vi "Lab Panel V5.28.vi"() -> ()   [LabVIEW 2013] (continued)
                                n843 = Unbundle(w1484) -> ("DESCRIPTION"=w1483:string)  [unwired: 4 out]
                                n844 = Concatenate Strings(w1479, "\\", w1477, w1475, w1476, w1475) -> (w1486:string)
                                n845 = String To Path(string=w1486) -> (path=w1488:path)
                                n846 = Concatenate Strings(w1486, w1485, w1483, "-", w1482, ".tdms") -> (w1474:string)
                                n847 = Create Folder(path (use dialog)=w1488) -> (error out=w1487:errorcluster)  [unwired: 2 in, 2 out]
                                n848 = global write "Global 1.vi" "LAB03-2 FILE"(w1474) -> ()
                                n849 = call <vilib>:"Clear Errors.vi"("error in (no error)"=w1487) -> ()  [unwired: 6 in, 1 out]
                              }
                              frame #1 {
                                (unwired) FALSE
                                n850 = String To Path(string=w1498) -> (path=w1494:path)
                                n851 = TDMS Open(6:FALSE, 10:T21."create or replace" ("operation (0:open)"), 11:w1494) -> (0:w1493:errorcluster, 3:→"TDMS LAB03-2":refnum<k34>)  [unwired: 4 in]
                              }
                              frame #2 {
                                n852 = local read "SET LAB03-2"() -> (w1504:T5)
                                n853 = local read "TDMS LAB03-2"() -> (w1515:refnum<k34>)
                                n854 = Build Array("Testers Name", "Description", "Set Test Cycles", "T-Rise minutes", "T-Rise Deg C") -> (w1505:string[])
                                n855 = Unbundle(w1504) -> ("NAME"=w1503:string, "DESCRIPTION"=w1502:string, "CYCLES"=w1501:dbl, "T-RISE mins"=w1500:dbl, "T-RISE deg C"=w1499:dbl)
                                n856 = Number To Decimal String(number=w1501) -> (decimal integer string=w1514:string)  [unwired: 1 in]
                                n857 = Number To Decimal String(number=w1500) -> (decimal integer string=w1513:string)  [unwired: 1 in]
                                n858 = Number To Decimal String(number=w1499) -> (decimal integer string=w1512:string)  [unwired: 1 in]
                                n859 = Build Array(w1503, w1502, w1514, w1513, w1512) -> (w1511:string[])
                                n860 = TDMS Set Properties(5:w1511, 7:w1505, 11:w1515) -> ()  [unwired: 3 in, 4 out]
                              }
                              frame #3 {
                                n861 = local read "DISP LAB03-2"() -> (w1520:T4)
                                n862 = Concatenate Strings("LAB03-2  ", w1519) -> (w1521:string)
                                n863 = Two Button Dialog(message=w1521, 1:w1517, 2:w1518) -> (T button?=w1523:bool)
                                n864 = case shown="True" w1523 {
                                tunnel: w1520 -> [w1530 w1531]
                                tunnel: [w1530 w1531] -> w1527
                                tunnel: [w1529 w1532] -> w1526
                                tunnel: [w1528 w1532] -> w1525
                                frame False {
                                n865 = Unbundle(w1530) -> ("CYCLE"=w1529:dbl, "MINS"=w1528:dbl)  [unwired: 1 out]
                                }
                                frame True {
                                w1532 = 0.0
                                }
                                }
                                n866 = Bundle(cluster=w1527, "CYCLE"=w1526, "MINS"=w1525, "STATUS"="RUN") -> (w1516:T4)
                                n867 = local write "DISP LAB03-2"(w1516) -> ()
                              }
                              frame #4 {
                                n868 = local read "TEMP START LAB03-2"() -> (w1535:cluster{"TL":dbl, "TN":dbl})
                                n869 = Bundle(cluster=w1535, "TL"=w1533, "TN"=w1533) -> (w1534:cluster{"TL":dbl, "TN":dbl})
                                n870 = local write "TEMP START LAB03-2"(w1534) -> ()
                              }
                            }
                          }
                        }
                      }
                    }
                  }
                }
              }
              event "RUN LAB04-1": Value Change {
                n871 = event-data() -> ("NewVal"=w1540:bool)  [unwired: 1 in, 5 out]
                n872 = local write "run lab04-1"(w1540) -> ()
                n873 = case shown="True" w1540 {
                  tunnel: w1546 -> [_ w1584]
                  tunnel: w1545 -> [_ w1583]
                  tunnel: w1543 -> [w1548 w1582]
                  tunnel: w1544 -> [_ w1581]
                  tunnel: w1542 -> [_ w1580]
                  tunnel: [w1547 w1579] -> w1541
                  tunnel: w1539 -> [_ w1578]
                  tunnel: w1538 -> [_ w1577]
                  tunnel: w1537 -> [_ w1576]
                  tunnel: w1536 -> [_ w1574]
                  frame False {
                    # "stop test"
                    n874 = stacked-sequence {
                      tunnel: w1548 -> [w1557 _]
                      tunnel: [w1549 _] -> w1547
                      frame #0 {
                        n875 = local read "DISP LAB04-1"() -> (w1556:T4)
                        n876 = Unbundle(w1556) -> ("CYCLE"=w1554:dbl, "MINS"=w1555:dbl)  [unwired: 1 out]
                        n877 = case shown="\"CYCLE TEST\"" w1557 {
                          tunnel: w1555 -> [_ _ w1564]
                          tunnel: w1554 -> [w1562 w1563 _]
                          tunnel: [w1562 w1563 w1564] -> w1553
                          frame "CHART TEST", Default {
                          }
                          frame "CYCLE TEST" {
                          }
                          frame "T-RISE TEST" {
                          }
                        }
                        n878 = local read "TDMS LAB04-1"() -> (w1561:refnum<k34>)
                        n879 = Build Array("STOPPED") -> (w1558:string[])
                        n880 = Build Array(w1553) -> (w1552:dbl[])
                        n881 = TDMS Write(0:w1561, 5:"TEST RESULT", 7:w1558, 9:w1552) -> (4:w1550:refnum<k34>, 15:w1551:errorcluster)  [unwired: 2 in, 2 out]
                        n882 = TDMS Close(8:w1551, 11:w1550) -> (0:w1549:errorcluster)  [unwired: 1 out]
                      }
                      frame #1 {
                        n883 = local read "DISP LAB04-1"() -> (w1568:T4)
                        n884 = stacked-sequence {
                          tunnel: "LAB04-1" -> [w1570 w1572]
                          frame #0 {
                            n885 = call "sub vi - defrag tdms v1.vi"("panel id"=w1570) -> ("error out"=w1569:errorcluster)  [unwired: 10 in]
                            n886 = local write "data file error"(w1569) -> ()
                          }
                          frame #1 {
                            n887 = call "Save data file (stop) v3.vi"("panel id"=w1572) -> ("network file save error"=w1571:errorcluster)  [unwired: 9 in, 1 out]
                            n888 = local write "RESULT LAB04-1"(FALSE) -> ()
                            n889 = local write "data file error"(w1571) -> ()
                          }
                        }
                        n890 = Bundle(cluster=w1568, "STATUS"="STOP") -> (w1566:T4)  [unwired: 2 in]
                        n891 = local write "DISP LAB04-1"(w1566) -> ()
                      }
                    }
                  }
                  frame True {
                    n892 = local read "SIG LAB04-1"() -> (w1575:T2)
                    n893 = stacked-sequence {
                      seq-local: [w1586 _] -> [_ w1590]
                      tunnel: w1584 -> [_ w1600]
                      tunnel: w1583 -> [_ w1599]
                      tunnel: w1582 -> [_ w1598]
                      tunnel: w1581 -> [_ w1597]
                      tunnel: w1580 -> [_ w1596]
                      tunnel: [_ w1595] -> w1579
                      tunnel: w1578 -> [_ w1594]
                      tunnel: w1577 -> [_ w1593]
                      tunnel: w1576 -> [_ w1592]
                      tunnel: w1575 -> [w1585 w1591]
                      tunnel: w1574 -> [_ w1589]
                      frame #0 {
                        n894 = Unbundle(w1585) -> ("AMPS"=w1588:dbl)  [unwired: 4 out]
                        n895 = call "Check For Amps on v1.vi"("ID"="LAB04-1", "amps"=w1588) -> ("amps"=w1586:bool)  [unwired: 9 in]
                      }
                      frame #1 {
                        n896 = case shown="True" w1590 {
                          tunnel: w1600 -> [_ w1613]
                          tunnel: w1599 -> [_ w1612]
                          tunnel: w1598 -> [_ w1611]
                          tunnel: w1597 -> [_ w1610]
                          tunnel: w1596 -> [_ w1609]
                          tunnel: [errorcluster {"status"=FALSE, "code"=0, "source"=""} ("error out") w1608] -> w1595
                          tunnel: w1594 -> [_ w1607]
                          tunnel: w1593 -> [_ w1606]
                          tunnel: w1592 -> [_ w1605]
                          tunnel: w1591 -> [_ w1604]
                          tunnel: w1589 -> [_ w1603]
                          frame False {
                            w1601 = FALSE
                            n897 = local write "RUN LAB04-1"(w1601) -> ()
                            n898 = local write "run lab04-1"(w1601) -> ()
                          }
                          frame True {
                            n899 = stacked-sequence {
                              seq-local: [w1614 _ _ _ _] -> [_ w1638 _ _ _]
                              tunnel: w1613 -> [w1619 _ _ _ _]
                              tunnel: w1612 -> [w1615 _ _ _ _]
                              tunnel: w1611 -> [w1629 _ _ _ _]
                              tunnel: w1610 -> [w1622 _ _ _ _]
                              tunnel: w1609 -> [w1617 _ _ _ _]
                              tunnel: [_ w1633 _ _ _] -> w1608
                              tunnel: w1607 -> [_ _ _ w1659 _]
                              tunnel: w1606 -> [_ _ _ w1658 _]
                              tunnel: w1605 -> [_ _ _ w1657 _]
                              tunnel: w1604 -> [_ _ _ _ _]
                              tunnel: w1603 -> [_ _ _ _ w1673]
                              frame #0 {
                                w1616 = "\\"
                                n900 = local read "SET LAB04-1"() -> (w1624:T5)
                                n901 = case shown="\"CYCLE TEST\"" w1629 {
                                tunnel: ["L04-1-CHART TEST-" "L04-1-CYCLE TEST-" "L04-1-T-RISE TEST-"] -> w1625
                                frame "CHART TEST", Default {
                                }
                                frame "CYCLE TEST" {
                                }
                                frame "T-RISE TEST" {
                                }
                                }
                                n902 = Unbundle(w1624) -> ("DESCRIPTION"=w1623:string)  [unwired: 4 out]
                                n903 = Concatenate Strings(w1619, "\\", w1617, w1616, w1615, w1616) -> (w1626:string)
                                n904 = String To Path(string=w1626) -> (path=w1628:path)
                                n905 = Concatenate Strings(w1626, w1625, w1623, "-", w1622, ".tdms") -> (w1614:string)
                                n906 = Create Folder(path (use dialog)=w1628) -> (error out=w1627:errorcluster)  [unwired: 2 in, 2 out]
                                n907 = global write "Global 1.vi" "LAB04-1 FILE"(w1614) -> ()
                                n908 = call <vilib>:"Clear Errors.vi"("error in (no error)"=w1627) -> ()  [unwired: 6 in, 1 out]
                              }
                              frame #1 {
                                (unwired) FALSE
                                n909 = String To Path(string=w1638) -> (path=w1634:path)
                                n910 = TDMS Open(6:FALSE, 10:T21."create or replace" ("operation (0:open)"), 11:w1634) -> (0:w1633:errorcluster, 3:→"TDMS LAB04-1":refnum<k34>)  [unwired: 4 in]
                              }
                              frame #2 {
                                n911 = local read "SET LAB04-1"() -> (w1644:T5)
                                n912 = local read "TDMS LAB04-1"() -> (w1655:refnum<k34>)
                                n913 = Build Array("Testers Name", "Description", "Set Test Cycles", "T-Rise minutes", "T-Rise Deg C") -> (w1645:string[])
                                n914 = Unbundle(w1644) -> ("NAME"=w1643:string, "DESCRIPTION"=w1642:string, "CYCLES"=w1641:dbl, "T-RISE mins"=w1640:dbl, "T-RISE deg C"=w1639:dbl)
                                n915 = Number To Decimal String(number=w1641) -> (decimal integer string=w1654:string)  [unwired: 1 in]
                                n916 = Number To Decimal String(number=w1640) -> (decimal integer string=w1653:string)  [unwired: 1 in]
                                n917 = Number To Decimal String(number=w1639) -> (decimal integer string=w1652:string)  [unwired: 1 in]
                                n918 = Build Array(w1643, w1642, w1654, w1653, w1652) -> (w1651:string[])
                                n919 = TDMS Set Properties(5:w1651, 7:w1645, 11:w1655) -> ()  [unwired: 3 in, 4 out]
                              }
                              frame #3 {
                                n920 = local read "DISP LAB04-1"() -> (w1660:T4)
                                n921 = Concatenate Strings("LAB04-1  ", w1659) -> (w1661:string)
                                n922 = Two Button Dialog(message=w1661, 1:w1657, 2:w1658) -> (T button?=w1663:bool)
                                n923 = case shown="True" w1663 {
                                tunnel: w1660 -> [w1670 w1671]
                                tunnel: [w1670 w1671] -> w1667
                                tunnel: [w1669 w1672] -> w1666
                                tunnel: [w1668 w1672] -> w1665
                                frame False {
                                n924 = Unbundle(w1670) -> ("CYCLE"=w1669:dbl, "MINS"=w1668:dbl)  [unwired: 1 out]
                                }
                                frame True {
                                w1672 = 0.0
                                }
                                }
                                n925 = Bundle(cluster=w1667, "CYCLE"=w1666, "MINS"=w1665, "STATUS"="RUN") -> (w1656:T4)
                                n926 = local write "DISP LAB04-1"(w1656) -> ()
                              }
                              frame #4 {
                                n927 = local read "TEMP START LAB04-1"() -> (w1675:cluster{"TL":dbl, "TN":dbl})
                                n928 = Bundle(cluster=w1675, "TL"=w1673, "TN"=w1673) -> (w1674:cluster{"TL":dbl, "TN":dbl})
                                n929 = local write "TEMP START LAB04-1"(w1674) -> ()
                              }
                            }
                          }
                        }
                      }
                    }
                  }
                }
              }
              event "RUN LAB04-2": Value Change {
                n930 = event-data() -> ("NewVal"=w1680:bool)  [unwired: 1 in, 5 out]
                n931 = local write "run lab04-2"(w1680) -> ()
                n932 = case shown="True" w1680 {
                  tunnel: w1686 -> [_ w1724]
                  tunnel: w1685 -> [_ w1723]
                  tunnel: w1683 -> [w1688 w1722]
                  tunnel: w1684 -> [_ w1721]
                  tunnel: w1682 -> [_ w1720]
                  tunnel: [w1687 w1719] -> w1681
                  tunnel: w1679 -> [_ w1718]
                  tunnel: w1678 -> [_ w1717]
                  tunnel: w1677 -> [_ w1716]
                  tunnel: w1676 -> [_ w1714]
                  frame False {
                    # "stop test"
                    n933 = stacked-sequence {
                      tunnel: w1688 -> [w1697 _]
                      tunnel: [w1689 _] -> w1687
                      frame #0 {
                        n934 = local read "DISP LAB04-2"() -> (w1696:T4)
                        n935 = Unbundle(w1696) -> ("CYCLE"=w1694:dbl, "MINS"=w1695:dbl)  [unwired: 1 out]
                        n936 = case shown="\"CYCLE TEST\"" w1697 {
                          tunnel: w1695 -> [_ _ w1704]
                          tunnel: w1694 -> [w1702 w1703 _]
                          tunnel: [w1702 w1703 w1704] -> w1693
                          frame "CHART TEST", Default {
                          }
                          frame "CYCLE TEST" {
                          }
                          frame "T-RISE TEST" {
                          }
                        }
                        n937 = local read "TDMS LAB04-2"() -> (w1701:refnum<k34>)
                        n938 = Build Array("STOPPED") -> (w1698:string[])
                        n939 = Build Array(w1693) -> (w1692:dbl[])
                        n940 = TDMS Write(0:w1701, 5:"TEST RESULT", 7:w1698, 9:w1692) -> (4:w1690:refnum<k34>, 15:w1691:errorcluster)  [unwired: 2 in, 2 out]
                        n941 = TDMS Close(8:w1691, 11:w1690) -> (0:w1689:errorcluster)  [unwired: 1 out]
                      }
                      frame #1 {
                        n942 = local read "DISP LAB04-2"() -> (w1708:T4)
                        n943 = stacked-sequence {
                          tunnel: "LAB04-2" -> [w1710 w1712]
                          frame #0 {
                            n944 = call "sub vi - defrag tdms v1.vi"("panel id"=w1710) -> ("error out"=w1709:errorcluster)  [unwired: 10 in]
                            n945 = local write "data file error"(w1709) -> ()
                          }
                          frame #1 {
                            n946 = call "Save data file (stop) v3.vi"("panel id"=w1712) -> ("network file save error"=w1711:errorcluster)  [unwired: 9 in, 1 out]
                            n947 = local write "RESULT LAB04-2"(FALSE) -> ()
                            n948 = local write "data file error"(w1711) -> ()
                          }
                        }
                        n949 = Bundle(cluster=w1708, "STATUS"="STOP") -> (w1706:T4)  [unwired: 2 in]
                        n950 = local write "DISP LAB04-2"(w1706) -> ()
                      }
                    }
                  }
                  frame True {
                    n951 = local read "SIG LAB04-2"() -> (w1715:T2)
                    n952 = stacked-sequence {
                      seq-local: [w1726 _] -> [_ w1730]
                      tunnel: w1724 -> [_ w1740]
                      tunnel: w1723 -> [_ w1739]
                      tunnel: w1722 -> [_ w1738]
                      tunnel: w1721 -> [_ w1737]
                      tunnel: w1720 -> [_ w1736]
                      tunnel: [_ w1735] -> w1719
                      tunnel: w1718 -> [_ w1734]
                      tunnel: w1717 -> [_ w1733]
                      tunnel: w1716 -> [_ w1732]
                      tunnel: w1715 -> [w1725 w1731]
                      tunnel: w1714 -> [_ w1729]
                      frame #0 {
                        n953 = Unbundle(w1725) -> ("AMPS"=w1728:dbl)  [unwired: 4 out]
                        n954 = call "Check For Amps on v1.vi"("ID"="LAB04-2", "amps"=w1728) -> ("amps"=w1726:bool)  [unwired: 9 in]
                      }
                      frame #1 {
                        n955 = case shown="True" w1730 {
                          tunnel: w1740 -> [_ w1753]
                          tunnel: w1739 -> [_ w1752]
                          tunnel: w1738 -> [_ w1751]
                          tunnel: w1737 -> [_ w1750]
                          tunnel: w1736 -> [_ w1749]
                          tunnel: [errorcluster {"status"=FALSE, "code"=0, "source"=""} ("error out") w1748] -> w1735
                          tunnel: w1734 -> [_ w1747]
                          tunnel: w1733 -> [_ w1746]
                          tunnel: w1732 -> [_ w1745]
                          tunnel: w1731 -> [_ w1744]
                          tunnel: w1729 -> [_ w1743]
                          frame False {
                            w1741 = FALSE
                            n956 = local write "RUN LAB04-2"(w1741) -> ()
                            n957 = local write "run lab04-2"(w1741) -> ()
                          }
                          frame True {
                            n958 = stacked-sequence {
                              seq-local: [w1754 _ _ _ _] -> [_ w1778 _ _ _]
                              tunnel: w1753 -> [w1759 _ _ _ _]
                              tunnel: w1752 -> [w1755 _ _ _ _]
                              tunnel: w1751 -> [w1769 _ _ _ _]
                              tunnel: w1750 -> [w1762 _ _ _ _]
                              tunnel: w1749 -> [w1757 _ _ _ _]
                              tunnel: [_ w1773 _ _ _] -> w1748
                              tunnel: w1747 -> [_ _ _ w1799 _]
                              tunnel: w1746 -> [_ _ _ w1798 _]
                              tunnel: w1745 -> [_ _ _ w1797 _]
                              tunnel: w1744 -> [_ _ _ _ _]
                              tunnel: w1743 -> [_ _ _ _ w1813]
                              frame #0 {
                                w1756 = "\\"
                                n959 = local read "SET LAB04-2"() -> (w1764:T5)
                                n960 = case shown="\"CHART TEST\", Default" w1769 {
                                tunnel: ["L04-2-CHART TEST-" "L04-2-CYCLE TEST-" "L04-2-T-RISE TEST-"] -> w1765
                                frame "CHART TEST", Default {
                                }
                                frame "CYCLE TEST" {
                                }
                                frame "T-RISE TEST" {
                                }
                                }
                                n961 = Unbundle(w1764) -> ("DESCRIPTION"=w1763:string)  [unwired: 4 out]
                                n962 = Concatenate Strings(w1759, "\\", w1757, w1756, w1755, w1756) -> (w1766:string)
                                n963 = String To Path(string=w1766) -> (path=w1768:path)
                                n964 = Concatenate Strings(w1766, w1765, w1763, "-", w1762, ".tdms") -> (w1754:string)
                                n965 = Create Folder(path (use dialog)=w1768) -> (error out=w1767:errorcluster)  [unwired: 2 in, 2 out]
                                n966 = global write "Global 1.vi" "LAB04-2 FILE"(w1754) -> ()
                                n967 = call <vilib>:"Clear Errors.vi"("error in (no error)"=w1767) -> ()  [unwired: 6 in, 1 out]
                              }
                              frame #1 {
                                (unwired) FALSE
                                n968 = String To Path(string=w1778) -> (path=w1774:path)
                                n969 = TDMS Open(6:FALSE, 10:T21."create or replace" ("operation (0:open)"), 11:w1774) -> (0:w1773:errorcluster, 3:→"TDMS LAB04-2":refnum<k34>)  [unwired: 4 in]
                              }
                              frame #2 {
                                n970 = local read "SET LAB04-2"() -> (w1784:T5)
                                n971 = local read "TDMS LAB04-2"() -> (w1795:refnum<k34>)
                                n972 = Build Array("Testers Name", "Description", "Set Test Cycles", "T-Rise minutes", "T-Rise Deg C") -> (w1785:string[])
                                n973 = Unbundle(w1784) -> ("NAME"=w1783:string, "DESCRIPTION"=w1782:string, "CYCLES"=w1781:dbl, "T-RISE mins"=w1780:dbl, "T-RISE deg C"=w1779:dbl)
                                n974 = Number To Decimal String(number=w1781) -> (decimal integer string=w1794:string)  [unwired: 1 in]
                                n975 = Number To Decimal String(number=w1780) -> (decimal integer string=w1793:string)  [unwired: 1 in]
                                n976 = Number To Decimal String(number=w1779) -> (decimal integer string=w1792:string)  [unwired: 1 in]
                                n977 = Build Array(w1783, w1782, w1794, w1793, w1792) -> (w1791:string[])
                                n978 = TDMS Set Properties(5:w1791, 7:w1785, 11:w1795) -> ()  [unwired: 3 in, 4 out]
                              }
                              frame #3 {
                                n979 = local read "DISP LAB04-2"() -> (w1800:T4)
                                n980 = Concatenate Strings("LAB04-2 ", w1799) -> (w1801:string)
                                n981 = Two Button Dialog(message=w1801, 1:w1797, 2:w1798) -> (T button?=w1803:bool)
                                n982 = case shown="True" w1803 {
                                tunnel: w1800 -> [w1810 w1811]
                                tunnel: [w1810 w1811] -> w1807
                                tunnel: [w1809 w1812] -> w1806
                                tunnel: [w1808 w1812] -> w1805
                                frame False {
                                n983 = Unbundle(w1810) -> ("CYCLE"=w1809:dbl, "MINS"=w1808:dbl)  [unwired: 1 out]
                                }
                                frame True {
                                w1812 = 0.0
                                }
                                }
                                n984 = Bundle(cluster=w1807, "CYCLE"=w1806, "MINS"=w1805, "STATUS"="RUN") -> (w1796:T4)
                                n985 = local write "DISP LAB04-2"(w1796) -> ()
                              }
                              frame #4 {
                                n986 = local read "TEMP START LAB04-2"() -> (w1815:cluster{"TL":dbl, "TN":dbl})
                                n987 = Bundle(cluster=w1815, "TL"=w1813, "TN"=w1813) -> (w1814:cluster{"TL":dbl, "TN":dbl})
                                n988 = local write "TEMP START LAB04-2"(w1814) -> ()
                              }
                            }
                          }
                        }
                      }
                    }
                  }
                }
              }
              event "RUN LAB05-1": Value Change {
                n989 = event-data() -> ("NewVal"=w1820:bool)  [unwired: 1 in, 5 out]
                n990 = local write "run lab05-1"(w1820) -> ()
                n991 = case shown="True" w1820 {
                  tunnel: w1826 -> [_ w1864]
                  tunnel: w1825 -> [_ w1863]
                  tunnel: w1823 -> [w1828 w1862]
                  tunnel: w1824 -> [_ w1861]
                  tunnel: w1822 -> [_ w1860]
                  tunnel: [w1827 w1859] -> w1821
                  tunnel: w1819 -> [_ w1858]
                  tunnel: w1818 -> [_ w1857]
                  tunnel: w1817 -> [_ w1856]
                  tunnel: w1816 -> [_ w1854]
                  frame False {
                    # "stop test"
                    n992 = stacked-sequence {
                      tunnel: w1828 -> [w1837 _]
                      tunnel: [w1829 _] -> w1827
                      frame #0 {
                        n993 = local read "DISP LAB05-1"() -> (w1836:T4)
                        n994 = Unbundle(w1836) -> ("CYCLE"=w1834:dbl, "MINS"=w1835:dbl)  [unwired: 1 out]
                        n995 = case shown="\"CYCLE TEST\"" w1837 {
                          tunnel: w1835 -> [_ _ w1844]
                          tunnel: w1834 -> [w1842 w1843 _]
                          tunnel: [w1842 w1843 w1844] -> w1833
                          frame "CHART TEST", Default {
                          }
                          frame "CYCLE TEST" {
                          }
                          frame "T-RISE TEST" {
                          }
                        }
                        n996 = local read "TDMS LAB05-1"() -> (w1841:refnum<k34>)
                        n997 = Build Array("STOPPED") -> (w1838:string[])
                        n998 = Build Array(w1833) -> (w1832:dbl[])
                        n999 = TDMS Write(0:w1841, 5:"TEST RESULT", 7:w1838, 9:w1832) -> (4:w1830:refnum<k34>, 15:w1831:errorcluster)  [unwired: 2 in, 2 out]
                        n1000 = TDMS Close(8:w1831, 11:w1830) -> (0:w1829:errorcluster)  [unwired: 1 out]
                      }
                      frame #1 {
                        n1001 = local read "DISP LAB05-1"() -> (w1848:T4)
                        n1002 = stacked-sequence {
                          tunnel: "LAB05-1" -> [w1850 w1852]
                          frame #0 {
                            n1003 = call "sub vi - defrag tdms v1.vi"("panel id"=w1850) -> ("error out"=w1849:errorcluster)  [unwired: 10 in]
                            n1004 = local write "data file error"(w1849) -> ()
                          }
                          frame #1 {
                            n1005 = call "Save data file (stop) v3.vi"("panel id"=w1852) -> ("network file save error"=w1851:errorcluster)  [unwired: 9 in, 1 out]
                            n1006 = local write "RESULT LAB05-1"(FALSE) -> ()
                            n1007 = local write "data file error"(w1851) -> ()
                          }
                        }
                        n1008 = Bundle(cluster=w1848, "STATUS"="STOP") -> (w1846:T4)  [unwired: 2 in]
                        n1009 = local write "DISP LAB05-1"(w1846) -> ()
                      }
                    }
                  }
                  frame True {
                    n1010 = local read "SIG LAB05-1"() -> (w1855:T2)
                    n1011 = stacked-sequence {
                      seq-local: [w1866 _] -> [_ w1870]
                      tunnel: w1864 -> [_ w1880]
                      tunnel: w1863 -> [_ w1879]
                      tunnel: w1862 -> [_ w1878]
                      tunnel: w1861 -> [_ w1877]
                      tunnel: w1860 -> [_ w1876]
                      tunnel: [_ w1875] -> w1859
                      tunnel: w1858 -> [_ w1874]
                      tunnel: w1857 -> [_ w1873]
                      tunnel: w1856 -> [_ w1872]
                      tunnel: w1855 -> [w1865 w1871]
                      tunnel: w1854 -> [_ w1869]
                      frame #0 {
                        n1012 = Unbundle(w1865) -> ("AMPS"=w1868:dbl)  [unwired: 4 out]
                        n1013 = call "Check For Amps on v1.vi"("ID"="LAB05-1", "amps"=w1868) -> ("amps"=w1866:bool)  [unwired: 9 in]
                      }
                      frame #1 {
                        n1014 = case shown="True" w1870 {
                          tunnel: w1880 -> [_ w1893]
                          tunnel: w1879 -> [_ w1892]
                          tunnel: w1878 -> [_ w1891]
                          tunnel: w1877 -> [_ w1890]
                          tunnel: w1876 -> [_ w1889]
                          tunnel: [errorcluster {"status"=FALSE, "code"=0, "source"=""} ("error out") w1888] -> w1875
                          tunnel: w1874 -> [_ w1887]
                          tunnel: w1873 -> [_ w1886]
                          tunnel: w1872 -> [_ w1885]
                          tunnel: w1871 -> [_ w1884]
                          tunnel: w1869 -> [_ w1883]
                          frame False {
                            w1881 = FALSE
                            n1015 = local write "RUN LAB05-1"(w1881) -> ()
                            n1016 = local write "run lab05-1"(w1881) -> ()
                          }
                          frame True {
                            n1017 = stacked-sequence {
                              seq-local: [w1894 _ _ _ _] -> [_ w1918 _ _ _]
                              tunnel: w1893 -> [w1899 _ _ _ _]
                              tunnel: w1892 -> [w1895 _ _ _ _]
                              tunnel: w1891 -> [w1909 _ _ _ _]
                              tunnel: w1890 -> [w1902 _ _ _ _]
                              tunnel: w1889 -> [w1897 _ _ _ _]
                              tunnel: [_ w1913 _ _ _] -> w1888
                              tunnel: w1887 -> [_ _ _ w1938 _]
                              tunnel: w1886 -> [_ _ _ w1937 _]
                              tunnel: w1885 -> [_ _ _ w1936 _]
                              tunnel: w1884 -> [_ _ _ _ _]
                              tunnel: w1883 -> [_ _ _ _ w1953]
                              frame #0 {
                                w1896 = "\\"
                                n1018 = local read "SET LAB05-1"() -> (w1904:T5)
                                n1019 = case shown="\"CYCLE TEST\"" w1909 {
                                tunnel: ["L05-1-CHART TEST-" "L05-1-CYCLE TEST-" "L05-1-T-RISE TEST-"] -> w1905
                                frame "CHART TEST", Default {
                                }
                                frame "CYCLE TEST" {
                                }
                                frame "T-RISE TEST" {
                                }
                                }
                                n1020 = Unbundle(w1904) -> ("DESCRIPTION"=w1903:string)  [unwired: 4 out]
                                n1021 = Concatenate Strings(w1899, "\\", w1897, w1896, w1895, w1896) -> (w1906:string)
                                n1022 = String To Path(string=w1906) -> (path=w1908:path)
                                n1023 = Concatenate Strings(w1906, w1905, w1903, "-", w1902, ".tdms") -> (w1894:string)
                                n1024 = Create Folder(path (use dialog)=w1908) -> (error out=w1907:errorcluster)  [unwired: 2 in, 2 out]
                                n1025 = global write "Global 1.vi" "LAB05-1 FILE"(w1894) -> ()
                                n1026 = call <vilib>:"Clear Errors.vi"("error in (no error)"=w1907) -> ()  [unwired: 6 in, 1 out]
                              }
                              frame #1 {
                                (unwired) FALSE
                                n1027 = String To Path(string=w1918) -> (path=w1914:path)
                                n1028 = TDMS Open(6:FALSE, 10:T21."create or replace" ("operation (0:open)"), 11:w1914) -> (0:w1913:errorcluster, 3:→"TDMS LAB05-1":refnum<k34>)  [unwired: 4 in]
                              }
                              frame #2 {
                                n1029 = local read "SET LAB05-1"() -> (w1924:T5)
                                n1030 = local read "TDMS LAB05-1"() -> (w1935:refnum<k34>)
                                n1031 = Build Array("Testers Name", "Description", "Set Test Cycles", "T-Rise minutes", "T-Rise Deg C") -> (w1925:string[])
                                n1032 = Unbundle(w1924) -> ("NAME"=w1923:string, "DESCRIPTION"=w1922:string, "CYCLES"=w1921:dbl, "T-RISE mins"=w1920:dbl, "T-RISE deg C"=w1919:dbl)
                                n1033 = Number To Decimal String(number=w1921) -> (decimal integer string=w1934:string)  [unwired: 1 in]
                                n1034 = Number To Decimal String(number=w1920) -> (decimal integer string=w1933:string)  [unwired: 1 in]
                                n1035 = Number To Decimal String(number=w1919) -> (decimal integer string=w1932:string)  [unwired: 1 in]
                                n1036 = Build Array(w1923, w1922, w1934, w1933, w1932) -> (w1931:string[])
                                n1037 = TDMS Set Properties(5:w1931, 7:w1925, 11:w1935) -> ()  [unwired: 3 in, 4 out]
                              }
                              frame #3 {
                                n1038 = local read "DISP LAB05-1"() -> (w1940:T4)
                                n1039 = Concatenate Strings("LAB05-1  ", w1938) -> (w1941:string)
                                n1040 = Two Button Dialog(message=w1941, 1:w1936, 2:w1937) -> (T button?=w1943:bool)
                                n1041 = case shown="True" w1943 {
                                tunnel: w1940 -> [w1950 w1951]
                                tunnel: [w1950 w1951] -> w1947
                                tunnel: [w1949 w1952] -> w1946
                                tunnel: [w1948 w1952] -> w1945
                                frame False {
                                n1042 = Unbundle(w1950) -> ("CYCLE"=w1949:dbl, "MINS"=w1948:dbl)  [unwired: 1 out]
                                }
                                frame True {
                                w1952 = 0.0
                                }
                                }
                                n1043 = Bundle(cluster=w1947, "CYCLE"=w1946, "MINS"=w1945, "STATUS"="RUN") -> (w1939:T4)
                                n1044 = local write "DISP LAB05-1"(w1939) -> ()
                              }
                              frame #4 {
                                n1045 = local read "TEMP START LAB05-1"() -> (w1955:cluster{"TL":dbl, "TN":dbl})
                                n1046 = Bundle(cluster=w1955, "TL"=w1953, "TN"=w1953) -> (w1954:cluster{"TL":dbl, "TN":dbl})
                                n1047 = local write "TEMP START LAB05-1"(w1954) -> ()
                              }
                            }
                          }
                        }
                      }
                    }
                  }
                }
              }
              event "RUN LAB05-2": Value Change {
                n1048 = event-data() -> ("NewVal"=w1961:bool)  [unwired: 1 in, 5 out]
                n1049 = local read "SIG LAB05-2"() -> (w1957:T2)
                n1050 = case shown="True" w1961 {
                  tunnel: w1967 -> [_ w2005]
                  tunnel: w1966 -> [_ w2004]
                  tunnel: w1964 -> [w1969 w2003]
                  tunnel: w1965 -> [_ w2002]
                  tunnel: w1963 -> [_ w2001]
                  tunnel: [w1968 w2000] -> w1962
                  tunnel: w1960 -> [_ w1999]
                  tunnel: w1959 -> [_ w1998]
                  tunnel: w1958 -> [_ w1997]
                  tunnel: w1957 -> [_ w1996]
                  tunnel: w1956 -> [_ w1995]
                  frame False {
                    # "stop test"
                    n1051 = stacked-sequence {
                      tunnel: w1969 -> [w1978 _]
                      tunnel: [w1970 _] -> w1968
                      frame #0 {
                        n1052 = local read "DISP LAB05-2"() -> (w1977:T4)
                        n1053 = Unbundle(w1977) -> ("CYCLE"=w1975:dbl, "MINS"=w1976:dbl)  [unwired: 1 out]
                        n1054 = case shown="\"CYCLE TEST\"" w1978 {
                          tunnel: w1976 -> [_ _ w1985]
                          tunnel: w1975 -> [w1983 w1984 _]
                          tunnel: [w1983 w1984 w1985] -> w1974
                          frame "CHART TEST", Default {
                          }
                          frame "CYCLE TEST" {
                          }
                          frame "T-RISE TEST" {
                          }
                        }
                        n1055 = local read "TDMS LAB05-2"() -> (w1982:refnum<k34>)
                        n1056 = Build Array("STOPPED") -> (w1979:string[])
                        n1057 = Build Array(w1974) -> (w1973:dbl[])
                        n1058 = TDMS Write(0:w1982, 5:"TEST RESULT", 7:w1979, 9:w1973) -> (4:w1971:refnum<k34>, 15:w1972:errorcluster)  [unwired: 2 in, 2 out]
                        n1059 = TDMS Close(8:w1972, 11:w1971) -> (0:w1970:errorcluster)  [unwired: 1 out]
                      }
                      frame #1 {
                        n1060 = local read "DISP LAB05-2"() -> (w1989:T4)
                        n1061 = stacked-sequence {
                          tunnel: "LAB05-2" -> [w1991 w1993]
                          frame #0 {
                            n1062 = call "sub vi - defrag tdms v1.vi"("panel id"=w1991) -> ("error out"=w1990:errorcluster)  [unwired: 10 in]
                            n1063 = local write "data file error"(w1990) -> ()
                          }
                          frame #1 {
                            n1064 = local write "RESULT LAB05-2"(FALSE) -> ()
                            n1065 = call "Save data file (stop) v3.vi"("panel id"=w1993) -> ("network file save error"=w1992:errorcluster)  [unwired: 9 in, 1 out]
                            n1066 = local write "data file error"(w1992) -> ()
                          }
                        }
                        n1067 = Bundle(cluster=w1989, "STATUS"="STOP") -> (w1987:T4)  [unwired: 2 in]
                        n1068 = local write "DISP LAB05-2"(w1987) -> ()
                      }
                    }
                  }
                  frame True {
                    n1069 = stacked-sequence {
                      seq-local: [w2007 _] -> [_ w2011]
                      tunnel: w2005 -> [_ w2021]
                      tunnel: w2004 -> [_ w2020]
                      tunnel: w2003 -> [_ w2019]
                      tunnel: w2002 -> [_ w2018]
                      tunnel: w2001 -> [_ w2017]
                      tunnel: [_ w2016] -> w2000
                      tunnel: w1999 -> [_ w2015]
                      tunnel: w1998 -> [_ w2014]
                      tunnel: w1997 -> [_ w2013]
                      tunnel: w1996 -> [w2006 w2012]
                      tunnel: w1995 -> [_ w2010]
                      frame #0 {
                        n1070 = Unbundle(w2006) -> ("AMPS"=w2009:dbl)  [unwired: 4 out]
                        n1071 = call "Check For Amps on v1.vi"("ID"="LAB05-2", "amps"=w2009) -> ("amps"=w2007:bool)  [unwired: 9 in]
                      }
                      frame #1 {
                        n1072 = case shown="True" w2011 {
                          tunnel: w2021 -> [_ w2034]
                          tunnel: w2020 -> [_ w2033]
                          tunnel: w2019 -> [_ w2032]
                          tunnel: w2018 -> [_ w2031]
                          tunnel: w2017 -> [_ w2030]
                          tunnel: [errorcluster {"status"=FALSE, "code"=0, "source"=""} ("error out") w2029] -> w2016
                          tunnel: w2015 -> [_ w2028]
                          tunnel: w2014 -> [_ w2027]
                          tunnel: w2013 -> [_ w2026]
                          tunnel: w2012 -> [_ w2025]
                          tunnel: w2010 -> [_ w2024]
                          frame False {
                            w2022 = FALSE
                            n1073 = local write "RUN LAB05-2"(w2022) -> ()
                            n1074 = local write "run lab05-2"(w2022) -> ()
                          }
                          frame True {
                            n1075 = stacked-sequence {
                              seq-local: [w2035 _ _ _ _] -> [_ w2059 _ _ _]
                              tunnel: w2034 -> [w2040 _ _ _ _]
                              tunnel: w2033 -> [w2036 _ _ _ _]
                              tunnel: w2032 -> [w2050 _ _ _ _]
                              tunnel: w2031 -> [w2043 _ _ _ _]
                              tunnel: w2030 -> [w2038 _ _ _ _]
                              tunnel: [_ w2054 _ _ _] -> w2029
                              tunnel: w2028 -> [_ _ _ w2079 _]
                              tunnel: w2027 -> [_ _ _ w2078 _]
                              tunnel: w2026 -> [_ _ _ w2077 _]
                              tunnel: w2025 -> [_ _ _ _ _]
                              tunnel: w2024 -> [_ _ _ _ w2094]
                              frame #0 {
                                w2037 = "\\"
                                n1076 = local read "SET LAB05-2"() -> (w2045:T5)
                                n1077 = case shown="\"CYCLE TEST\"" w2050 {
                                tunnel: ["L05-2-CHART TEST-" "L05-2-CYCLE TEST-" "L05-2-T-RISE TEST-"] -> w2046
                                frame "CHART TEST", Default {
                                }
                                frame "CYCLE TEST" {
                                }
                                frame "T-RISE TEST" {
                                }
                                }
                                n1078 = Unbundle(w2045) -> ("DESCRIPTION"=w2044:string)  [unwired: 4 out]
                                n1079 = Concatenate Strings(w2040, "\\", w2038, w2037, w2036, w2037) -> (w2047:string)
                                n1080 = String To Path(string=w2047) -> (path=w2049:path)
                                n1081 = Concatenate Strings(w2047, w2046, w2044, "-", w2043, ".tdms") -> (w2035:string)
                                n1082 = Create Folder(path (use dialog)=w2049) -> (error out=w2048:errorcluster)  [unwired: 2 in, 2 out]
                                n1083 = global write "Global 1.vi" "LAB05-2 FILE"(w2035) -> ()
                                n1084 = call <vilib>:"Clear Errors.vi"("error in (no error)"=w2048) -> ()  [unwired: 6 in, 1 out]
                              }
                              frame #1 {
                                (unwired) FALSE
                                n1085 = String To Path(string=w2059) -> (path=w2055:path)
                                n1086 = TDMS Open(6:FALSE, 10:T21."create or replace" ("operation (0:open)"), 11:w2055) -> (0:w2054:errorcluster, 3:→"TDMS LAB05-2":refnum<k34>)  [unwired: 4 in]
                              }
                              frame #2 {
                                n1087 = local read "SET LAB05-2"() -> (w2065:T5)
                                n1088 = local read "TDMS LAB05-2"() -> (w2076:refnum<k34>)
                                n1089 = Build Array("Testers Name", "Description", "Set Test Cycles", "T-Rise minutes", "T-Rise Deg C") -> (w2066:string[])
                                n1090 = Unbundle(w2065) -> ("NAME"=w2064:string, "DESCRIPTION"=w2063:string, "CYCLES"=w2062:dbl, "T-RISE mins"=w2061:dbl, "T-RISE deg C"=w2060:dbl)
                                n1091 = Number To Decimal String(number=w2062) -> (decimal integer string=w2075:string)  [unwired: 1 in]
                                n1092 = Number To Decimal String(number=w2061) -> (decimal integer string=w2074:string)  [unwired: 1 in]
                                n1093 = Number To Decimal String(number=w2060) -> (decimal integer string=w2073:string)  [unwired: 1 in]
                                n1094 = Build Array(w2064, w2063, w2075, w2074, w2073) -> (w2072:string[])
                                n1095 = TDMS Set Properties(5:w2072, 7:w2066, 11:w2076) -> ()  [unwired: 3 in, 4 out]
                              }
                              frame #3 {
                                n1096 = local read "DISP LAB05-2"() -> (w2081:T4)
                                n1097 = Concatenate Strings("LAB05-2  ", w2079) -> (w2082:string)
                                n1098 = Two Button Dialog(message=w2082, 1:w2077, 2:w2078) -> (T button?=w2084:bool)
                                n1099 = case shown="True" w2084 {
                                tunnel: w2081 -> [w2091 w2092]
                                tunnel: [w2091 w2092] -> w2088
                                tunnel: [w2090 w2093] -> w2087
                                tunnel: [w2089 w2093] -> w2086
                                frame False {
                                n1100 = Unbundle(w2091) -> ("CYCLE"=w2090:dbl, "MINS"=w2089:dbl)  [unwired: 1 out]
                                }
                                frame True {
                                w2093 = 0.0
                                }
                                }
                                n1101 = Bundle(cluster=w2088, "CYCLE"=w2087, "MINS"=w2086, "STATUS"="RUN") -> (w2080:T4)
                                n1102 = local write "DISP LAB05-2"(w2080) -> ()
                              }
                              frame #4 {
                                n1103 = local read "TEMP START LAB05-2"() -> (w2096:cluster{"TL":dbl, "TN":dbl})
                                n1104 = Bundle(cluster=w2096, "TL"=w2094, "TN"=w2094) -> (w2095:cluster{"TL":dbl, "TN":dbl})
                                n1105 = local write "TEMP START LAB05-2"(w2095) -> ()
                              }
                            }
                          }
                        }
                      }
                    }
                  }
                }
                n1106 = local write "run lab05-2"(w1961) -> ()
              }
            }
            n1107 = local write "data file error"(w665) -> ()
          }
          frame #5 {
            # "check if test cycles reached for cycle tests, if so then test pass"
            n1108 = stacked-sequence {
              tunnel: w2116 -> [_ _ _ _ _ _ _ _ _ _]
              tunnel: w2115 -> [_ _ _ _ _ _ _ _ _ _]
              tunnel: w2114 -> [_ _ _ _ _ _ _ _ _ _]
              tunnel: w2113 -> [_ _ _ _ _ _ _ _ _ _]
              tunnel: w2112 -> [_ _ _ _ _ _ _ _ _ _]
              tunnel: w2111 -> [_ _ _ _ _ _ _ _ _ _]
              tunnel: w2110 -> [_ _ _ _ _ _ _ _ _ _]
              tunnel: w2109 -> [_ _ _ _ _ _ _ _ _ _]
              tunnel: w2108 -> [_ _ _ _ _ _ _ _ _ _]
              tunnel: w2107 -> [_ _ _ _ _ _ _ _ _ _]
              tunnel: w2106 -> [w2122 _ _ _ _ _ _ _ _ _]
              tunnel: w2105 -> [_ w2157 _ _ _ _ _ _ _ _]
              tunnel: w2104 -> [_ _ w2197 _ _ _ _ _ _ _]
              tunnel: w2103 -> [_ _ _ w2237 _ _ _ _ _ _]
              tunnel: w2102 -> [_ _ _ _ w2277 _ _ _ _ _]
              tunnel: w2101 -> [_ _ _ _ _ w2317 _ _ _ _]
              tunnel: w2100 -> [_ _ _ _ _ _ w2357 _ _ _]
              tunnel: w2099 -> [_ _ _ _ _ _ _ w2397 _ _]
              tunnel: w2098 -> [_ _ _ _ _ _ _ _ w2437 _]
              tunnel: w2097 -> [_ _ _ _ _ _ _ _ _ w2477]
              frame #0 {
                # "LAB01-1"
                n1109 = Less?(x=w2122, y=2) -> (x < y?=w2120:bool)
                n1110 = local read "DISP LAB01-1"() -> (w2123:T4)
                n1111 = Unbundle(w2123) -> ("STATUS"=w2117:string)  [unwired: 2 out]
                n1112 = Equal?(x=w2117, y="RUN") -> (x = y?=w2119:bool)
                n1113 = And(x=w2119, y=w2120) -> (x .and. y?=w2118:bool)
                n1114 = case shown="True" w2118 {
                  tunnel: w2123 -> [_ w2128]
